vi "Create.vi"(8 "Error In":errorcluster, 11 "labssh2 Shared Library":path=path "") -> (0 "Error Out":errorcluster, 3 "Sesssion":refnum<class "Session.lvclass">)   [LabVIEW 2017, in "LabSSH2.lvlib" / "Session.lvclass"]
uses:
  Session.lvclass
  Session.lvclass/Session.ctl
  <vilib>/Utility/error.llb/Error Cluster From Error Code.vi
  <vilib>/ErrorRing/Error Ring.xnode
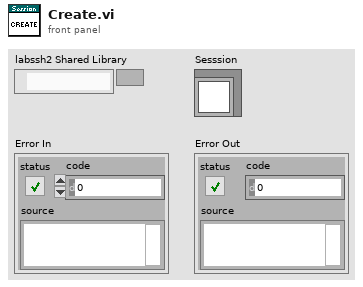
[diagram p1: front panel]
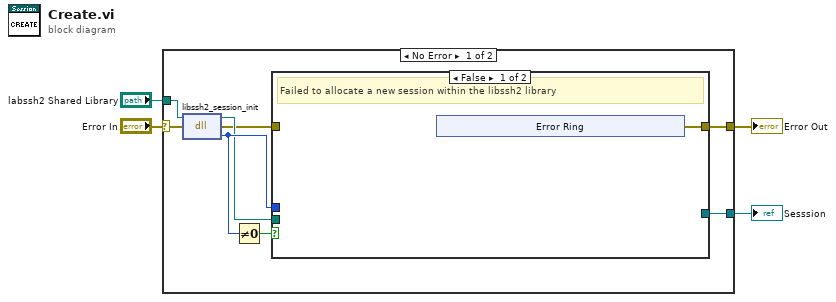
[diagram p0: block diagram]
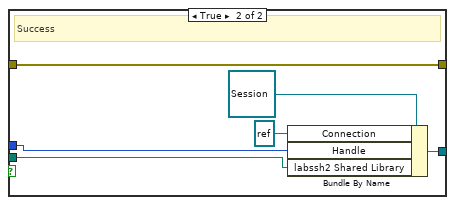
[diagram p2: hidden frame]
diagram:
  n1 = case shown="No Error" "Error In" {
    selector: "Error In" -> [w12 w24]
    tunnel: "labssh2 Shared Library" -> [w11 _]
    tunnel: [w5 w24] -> w2
    tunnel: [w7 _] -> w1
    frame No Error {
      n2 = dll-call lib="D:/Users/cfield/Code/Field R&D Services/SSH/LabSSH2/LabVIEW/trunk/src/LabSSH2/Private/labssh2.*" fn="libssh2_session_init"(path in=w11, error in=w12) -> (path out=w8:path, error out=w6:errorcluster, "SESSION"=w9:u64)  [unwired: 1 in]
      n3 = Not Equal To 0?(x=w9) -> (x != 0?=w10:bool)
      n4 = case shown="False" w10 {
        tunnel: w9 -> [_ w23]
        tunnel: w8 -> [_ w22]
        tunnel: [_ w21] -> w7
        tunnel: w6 -> [_ w18]
        tunnel: [w13 w18] -> w5
        frame False {
          # "Failed to allocate a new session within the libssh2 library"
          n5 = xnode "Error Ring"() -> ("error out"=w13:errorcluster)
        }
        frame True {
          # "Success"
          n6 = Bundle By Name(cluster=refnum<class "Session.lvclass"> refnum ("LabSSH2.lvlib:Session.lvclass"), "Connection"=refnum<k5> refnum, "Handle"=w23, "labssh2 Shared Library"=w22) -> (w21:refnum<class "Session.lvclass">)
        }
      }
    }
    frame Error {
    }
  }
  "Sesssion" <- w1
  "Error Out" <- w2
